vi "LinVer Protokoll_Daten.vi"(9 "Lin-Polynom":T4={"Messgerät"="", "Kalibrator (Gasteiler)"="", "Bearbeiter/in"="", "Komponente"="", "Zeitstempel"=timestamp(0 s since 1904-01-01), "F_max gefordert (%)"=0.0, "F_max in %"=0.0, "F_max in ppm"=0.0, "Vorschlag Ordnung"=0, "Polynom OK"=FALSE, "Polynomkoeff."=[], "Prüfgas Konzentration"=0.0, "Pfad EPA"="", "Pfad_LIN"="", "Gasnummer:"=0, "Komponentenauswahl"=[], "Verdünnungsgas"=0, "Zeitdauer Stufe"=0.0, "Anzahl Stufen"=0.0, "F_max in % EPA"=0.0, "F_max in ppm EPA"=0.0, "F_max in % LIN"=0.0, "F_max in ppm LIN"=0.0, "Punkte umkehren"=FALSE, "EPA Optionsfeld"=enum."Rohwert", "Autolin Hovacal"=enum."Optionsauswahl 2", "Spanfactors"=[], "Kalibrierauswahl"=0, "Conditions:"=0, "Gasflaschen Nr.:"="", "Bottle Accuracy"=0.0, "Konfig Gasflasche"=FALSE, "Gasflasche"=0, "HovaCAL Flow AutoLin"={"HovaCAL Flow Input Cluster"=0.0}, "MFC Output"={"Run"=FALSE}, "Gas Ablaufdatum"=timestamp(0 s since 1904-01-01), "Lin Modus"=0, "zusätzliche Zeitdauer Erster Punkt"=0.0, "Offsets"=[]} {"zusätzliche Zeitdauer Erster Punkt" format="%#_5g"; "Lin Modus" items=["Cal Gas to PNS", "Cal Gas to Samplepoint", "Measure"]; "Gas Ablaufdatum" format="%<%d.%m.%Y>T"; "HovaCAL Flow AutoLin"."HovaCAL Flow Input Cluster" format="%.2f"; "Gasflasche" items=["----"=10000, "IAG MG"=0, "IAG NH3 3000"=1, "IAG NH3 2000"=2, "IAG NH3 200"=3]; "Conditions:" items=["field", "laboratory"]; "Kalibrierauswahl" items=["Inaktiv", "Aktiv"]; "Anzahl Stufen" format="%#_5g"; "Zeitdauer Stufe" format="%#_5g"; "Verdünnungsgas" items=["N2", "O2"]; "Komponentenauswahl"."Konzentration" format="%#.6f"; "Gasnummer:" min=1 max=5; "Prüfgas Konzentration" format="%#.6f"; "Polynomkoeff." format="%#_18f"}, 10 "Aktiv":T1, 11 "Eingabetabelle":T3) -> (0 "EPA Auswertung":cluster{sgl[], sgl[], bool[]}, 1 "Ausgangs-Cluster":T4={"Messgerät"="", "Kalibrator (Gasteiler)"="", "Bearbeiter/in"="", "Komponente"="", "Zeitstempel"=timestamp(0 s since 1904-01-01), "F_max gefordert (%)"=0.0, "F_max in %"=0.0, "F_max in ppm"=0.0, "Vorschlag Ordnung"=0, "Polynom OK"=FALSE, "Polynomkoeff."=[], "Prüfgas Konzentration"=0.0, "Pfad EPA"="", "Pfad_LIN"="", "Gasnummer:"=0, "Komponentenauswahl"=[], "Verdünnungsgas"=0, "Zeitdauer Stufe"=0.0, "Anzahl Stufen"=0.0, "F_max in % EPA"=0.0, "F_max in ppm EPA"=0.0, "F_max in % LIN"=0.0, "F_max in ppm LIN"=0.0, "Punkte umkehren"=FALSE, "EPA Optionsfeld"=enum."Rohwert", "Autolin Hovacal"=enum."Optionsauswahl 2", "Spanfactors"=[], "Kalibrierauswahl"=0, "Conditions:"=0, "Gasflaschen Nr.:"="", "Bottle Accuracy"=0.0, "Konfig Gasflasche"=FALSE, "Gasflasche"=0, "HovaCAL Flow AutoLin"={"HovaCAL Flow Input Cluster"=0.0}, "MFC Output"={"Run"=FALSE}, "Gas Ablaufdatum"=timestamp(0 s since 1904-01-01), "Lin Modus"=0, "zusätzliche Zeitdauer Erster Punkt"=0.0, "Offsets"=[]} {"zusätzliche Zeitdauer Erster Punkt" format="%#_5g"; "Lin Modus" items=["Cal Gas to PNS", "Cal Gas to Samplepoint", "Measure"]; "Gas Ablaufdatum" format="%<%d.%m.%Y>T"; "HovaCAL Flow AutoLin"."HovaCAL Flow Input Cluster" format="%.2f"; "Gasflasche" items=["----"=10000, "IAG MG"=0, "IAG NH3 3000"=1, "IAG NH3 2000"=2, "IAG NH3 200"=3]; "Conditions:" items=["field", "laboratory"]; "Kalibrierauswahl" items=["Inaktiv", "Aktiv"]; "Anzahl Stufen" format="%#_5g"; "Zeitdauer Stufe" format="%#_5g"; "Verdünnungsgas" items=["N2", "O2"]; "Komponentenauswahl"."Konzentration" format="%#.6f"; "Gasnummer:" min=1 max=5; "Prüfgas Konzentration" format="%#.6f"; "Polynomkoeff." format="%#_18f"}, 2 "Auswertung Daten":string[](array[string]), 3 "Tabelle":T3)   [LabVIEW 2020, in "Linearisierung v2.lvlib" / "Linearity verification 1065-307.lvlib"]
uses:
  Linearity verification 1065-307.lvlib
  Lin-Polynom Daten.ctl
  KomponentenArray.ctl
  Visualisierungs Elemente/Auswahlfeld.ctl
  Visualisierungs Elemente/Zahlen-Eingabefeld.ctl
  EPA Optionsfeld.ctl
  Gasteiler/HovaCal/AutoLin Hovacal.ctl
  Kalibrieroption.ctl
  Condition.ctl
  Seiten/System Einstellungen V2/Konfig Gasflasche.ctl
  Seiten/System Einstellungen V2/Gasflasche Auswahl.ctl
  Gasteiler/HovaCAL_Interface/Controls/Flow Einstellung.ctl
  Gasteiler/HovaCAL_Interface/Controls/Pump state.ctl
  Seiten/CalGas Aufschaltung/Lin Modus.ctl
  Eingabetabelle.ctl
  AktivArray.ctl
  AktivButton.ctl
  Sprachverwaltung/FGV Aktion Tabelle zerlegen.ctl
  Sprachverwaltung/Sprachverwaltung.lvlib
  AutoLin Protokoll/AutoLin Protokoll.lvlib
  Linearisierung v2.lvlib
  Allgemein/allgemeine Sub-VIs.lvlib
  Gasteiler/Gasteiler.lvlib
  Gasteiler/HovaCal/HovaCal.lvlib
  Seiten/System Einstellungen V2/System Einstellungen V2.lvlib
  Gasteiler/HovaCAL_Interface/Controls/Controls.lvlib
  Seiten/CalGas Aufschaltung/CalGas Aufschaltung.lvlib
panel:
  # "Tabelle:\n0.....Sollwert\n1.....Istwert\n2.....Rohwert\n3.....linearisiert\n4.....abs.Fehler ppm\n5.....Fehler in %\n6.....Deviation\n7.....Temp.Messzelle\n8.....Druck Messzelle\n9.....abs.Fehler ppm linearisiert\n10....Fehler in % linearisiert\n11....abs.Fehler ppm EPA\n12....Fehler in % EPA\n13....abs.Fehler ppm Rohwert\n14....Fehler in % Rohwert"
  # "%"
  # "%"
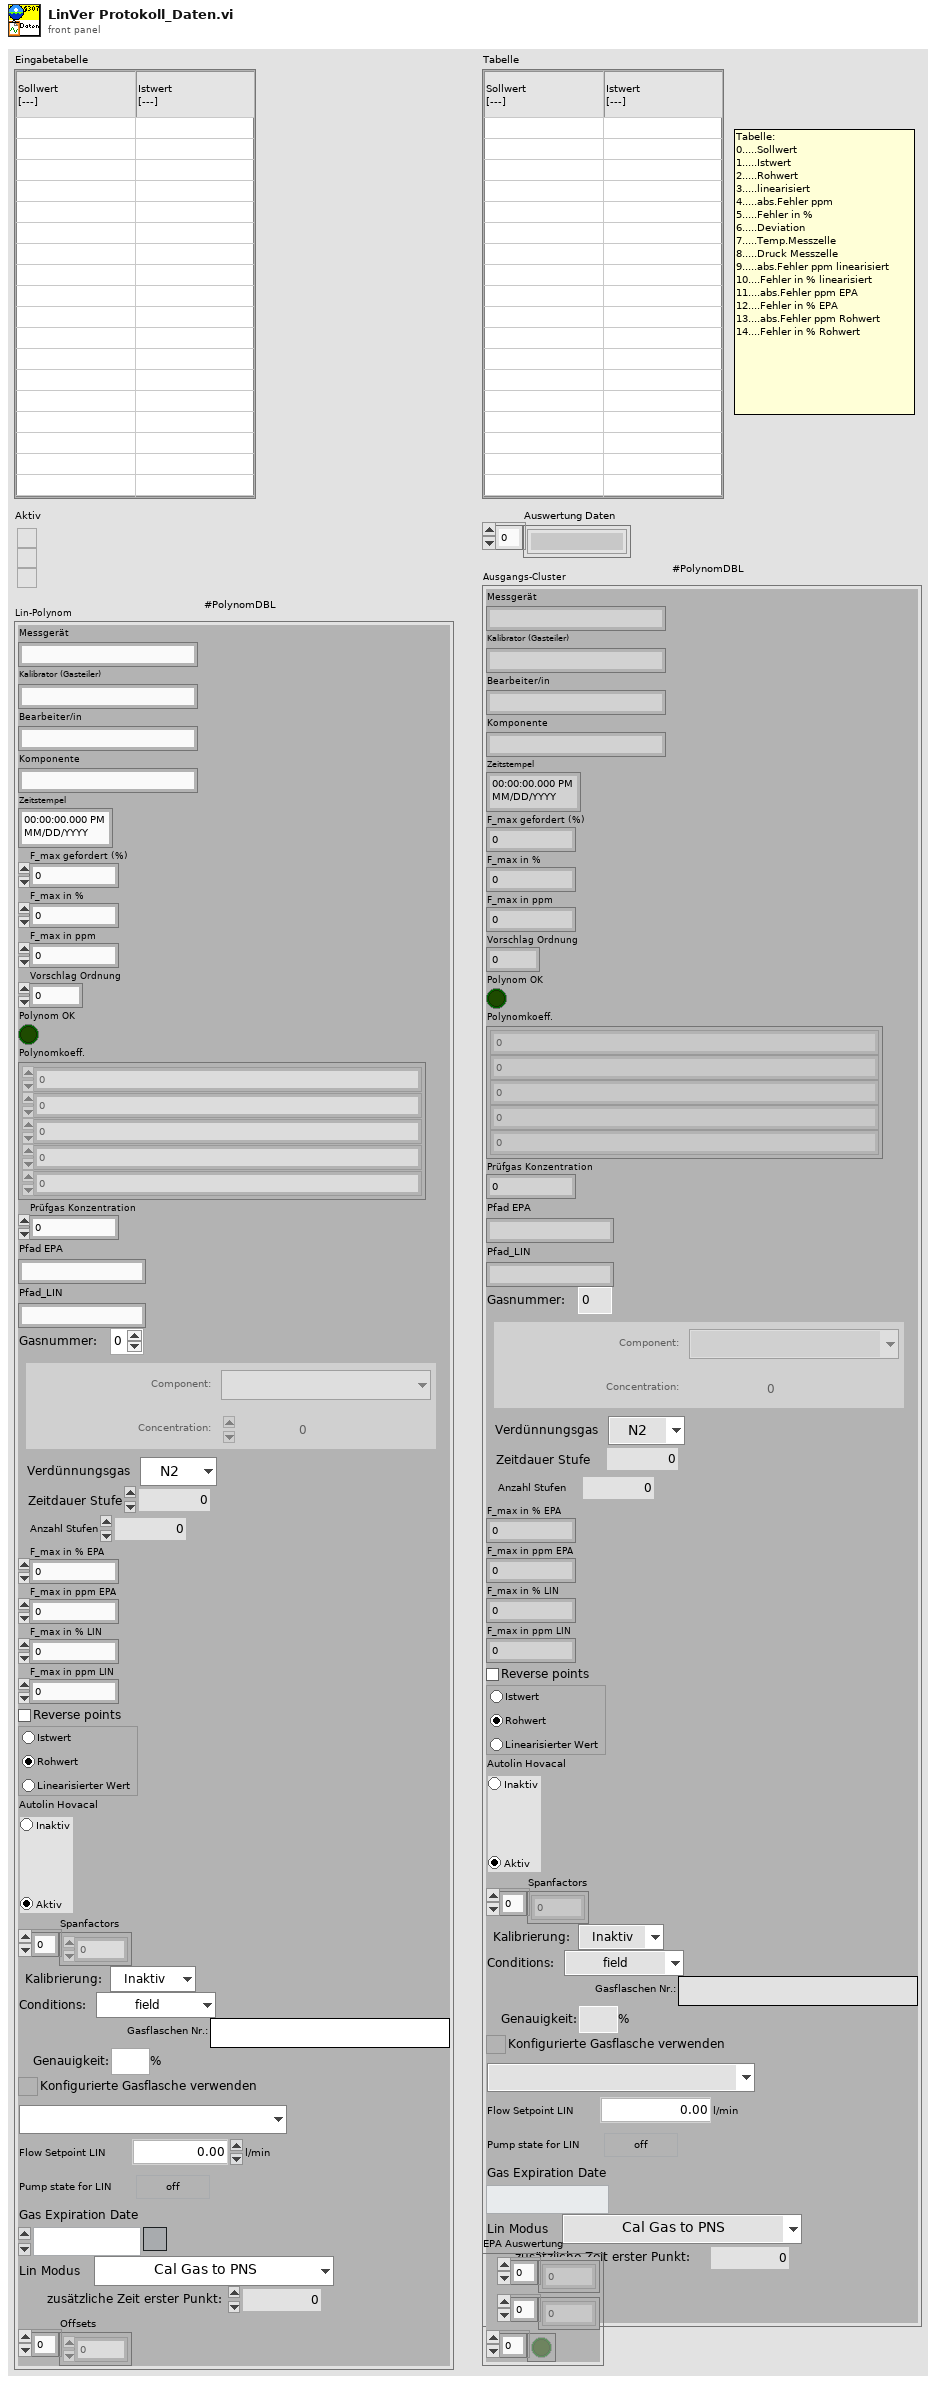
[diagram p1: front panel]
types:
  T1 = typedef "Linearisierung v2.lvlib/AktivArray.ctl" = T2[]
  T2 = typedef "Linearisierung v2.lvlib/AktivButton.ctl" = bool
  T3 = typedef "Linearisierung v2.lvlib/Eingabetabelle.ctl" = string[][]
  T4 = typedef "Linearisierung v2.lvlib/Lin-Polynom Daten.ctl" = cluster{"Messgerät":string, "Kalibrator (Gasteiler)":string, "Bearbeiter/in":string, "Komponente":string, "Zeitstempel":timestamp, "F_max gefordert (%)":sgl, "F_max in %":sgl, "F_max in ppm":sgl, "Vorschlag Ordnung":i32, "Polynom OK":bool, "Polynomkoeff.":dbl[], "Prüfgas Konzentration":dbl, "Pfad EPA":string, "Pfad_LIN":string, "Gasnummer:":u8, "Komponentenauswahl":T5, "Verdünnungsgas":T7, "Zeitdauer Stufe":T8, "Anzahl Stufen":T8, "F_max in % EPA":sgl, "F_max in ppm EPA":sgl, "F_max in % LIN":sgl, "F_max in ppm LIN":sgl, "Punkte umkehren":bool, "EPA Optionsfeld":T9, "Autolin Hovacal":T10, "Spanfactors":sgl[], "Kalibrierauswahl":T11, "Conditions:":T12, "Gasflaschen Nr.:":string, "Bottle Accuracy":dbl, "Konfig Gasflasche":T13, "Gasflasche":T14, "HovaCAL Flow AutoLin":T15, "MFC Output":T16, "Gas Ablaufdatum":timestamp, "Lin Modus":T17, "zusätzliche Zeitdauer Erster Punkt":sgl, "Offsets":sgl[]}
  T5 = typedef "Linearisierung v2.lvlib/KomponentenArray.ctl" = cluster{"Komponente:":T6, "Konzentration":dbl}[]
  T6 = typedef "Auswahlfeld.ctl" = u16
  T7 = typedef "Linearisierung v2.lvlib/Gasteiler.lvlib/Prüfgas in.ctl" = u16
  T8 = typedef "Zahlen-Eingabefeld.ctl" = sgl
  T9 = typedef "Linearisierung v2.lvlib/EPA Optionsfeld.ctl" = enum32{"Istwert", "Rohwert", "Linearisierter Wert"}
  T10 = typedef "Linearisierung v2.lvlib/Gasteiler.lvlib/HovaCal.lvlib/AutoLin Hovacal.ctl" = enum32{"Keine Auswahl", "Optionsauswahl 1", "Optionsauswahl 2"}
  T11 = typedef "Linearisierung v2.lvlib/Kalibrieroption.ctl" = u16
  T12 = typedef "Linearisierung v2.lvlib/Linearity verification 1065-307.lvlib/Condition.ctl" = u16
  T13 = typedef "System Einstellungen V2.lvlib/Konfig Gasflasche.ctl" = bool
  T14 = typedef "System Einstellungen V2.lvlib/Gasflasche Auswahl.ctl" = u16
  T15 = typedef "Linearisierung v2.lvlib/Gasteiler.lvlib/HovaCAL_Interface.lvlib/Controls.lvlib/Flow Einstellung.ctl" = cluster{"HovaCAL Flow Input Cluster":dbl}
  T16 = typedef "Linearisierung v2.lvlib/Gasteiler.lvlib/HovaCAL_Interface.lvlib/Controls.lvlib/Pump state.ctl" = cluster{"Run":bool}
  T17 = typedef "CalGas Aufschaltung.lvlib/Lin Modus.ctl" = u16
  T18 = typedef "Sprachverwaltung.lvlib/FGV Aktion Tabelle zerlegen.ctl" = enum16{"laden", "vereinzeln", "speichern"}
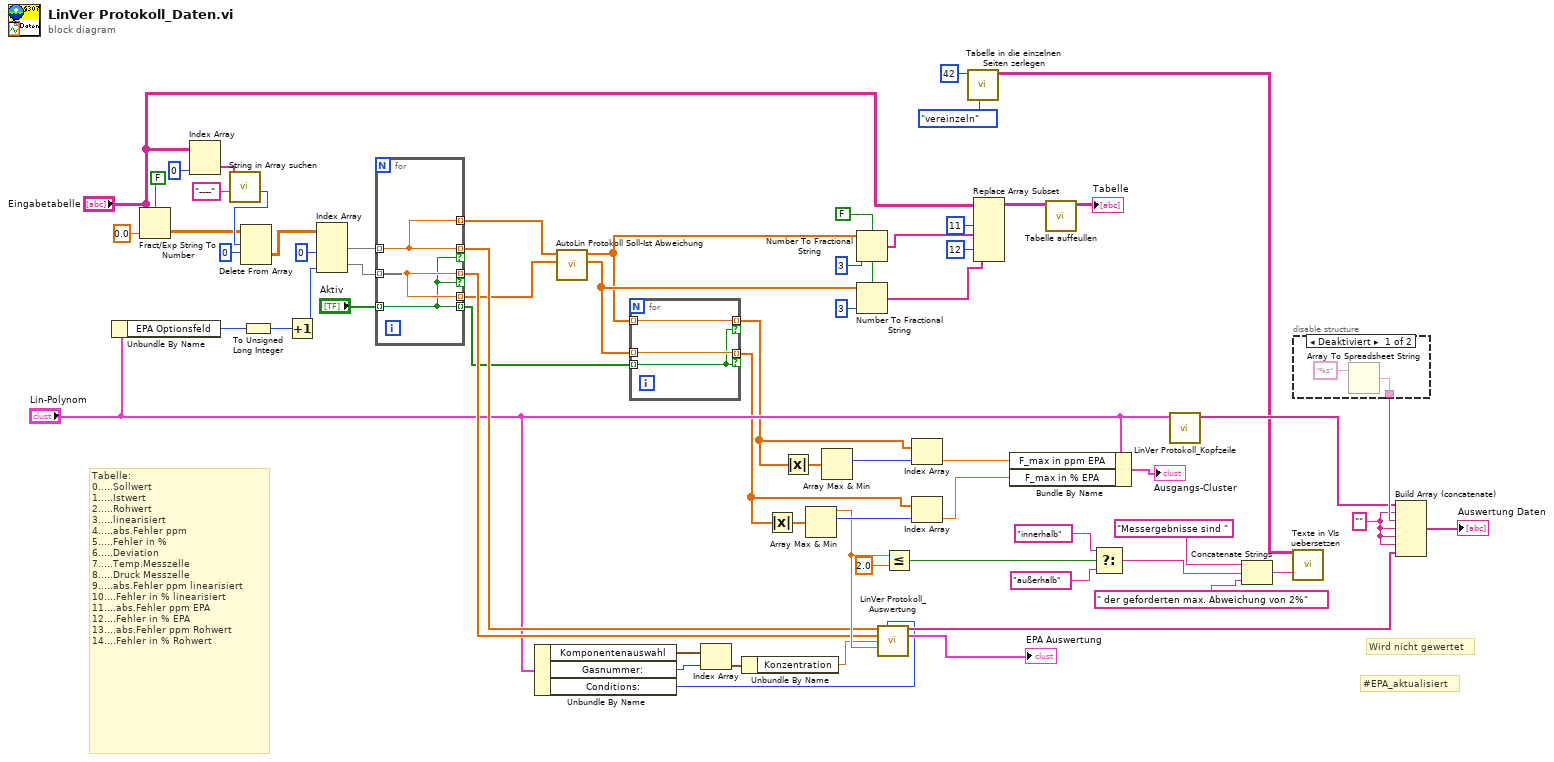
[diagram p0: block diagram]
diagram:
  w3 = FALSE ("Systemdezimalzeichen verwenden (T)")
  w44 = ""
  # "Tabelle:\n0.....Sollwert\n1.....Istwert\n2.....Rohwert\n3.....linearisiert\n4.....abs.Fehler ppm\n5.....Fehler in %\n6.....Deviation\n7.....Temp.Messzelle\n8.....Druck Messzelle\n9.....abs.Fehler ppm linearisiert\n10....Fehler in % linearisiert\n11....abs.Fehler ppm EPA\n12....Fehler in % EPA\n13....abs.Fehler ppm Rohwert\n14....Fehler in % Rohwert"
  # "#EPA_aktualisiert"
  # "Wird nicht gewertet"
  n1 = Unbundle By Name("Lin-Polynom") -> ("EPA Optionsfeld"=w13:T9)
  n2 = Fract/Exp String To Number(use system decimal point (T)=FALSE ("Systemdezimalzeichen verwenden (T)"), string="Eingabetabelle", default (0 dbl)=0.0) -> (number=w17:dbl[][])  [unwired: 1 in, 1 out]
  n3 = Index Array(array="Eingabetabelle", index (col)=0 ("Deaktivierter Index (Spalte)")) -> (element=w20:string[])  [unwired: 1 in]
  n4 = call "String in Array suchen.vi"("Nach String/Zeichen suchen (-)"="----", "String-Array"=w20) -> ("Index"=w21:i32)  [unwired: 7 in, 2 out]
  n5 = Delete From Array(array=w17, length=w21, index (row)=0 ("Index (Zeile)")) -> (deleted portion=w16:dbl[][])  [unwired: 1 in, 1 out]
  n6 = To Unsigned Long Integer(number=w13) -> (unsigned 32bit integer=w12:u32)
  n7 = Increment(x=w12) -> (x+1=w11:u32)
  n8 = Index Array(array=w16, index (col) #1=0 ("Deaktivierter Index (Spalte)"), index (col) #2=w11) -> (element #1=w30:dbl[], element #2=w29:dbl[])  [unwired: 2 in]
  n9 = for {
    tunnel: w30 -> [w69] mode=indexing
    tunnel: w29 -> [w68] mode=indexing
    tunnel: [w69] -> w27 mode=indexing if=w67
    tunnel: [w68] -> w26 mode=indexing if=w67
    tunnel: "Aktiv" -> [w67] mode=indexing
    tunnel: [w69] -> w10 mode=indexing
    tunnel: [w68] -> w9 mode=indexing
    tunnel: [w67] -> w7 mode=indexing
  }
  n10 = Unbundle By Name("Lin-Polynom") -> ("Komponentenauswahl"=w35:T5, "Gasnummer:"=w32:u8, "Conditions:"=w1:T12)
  n11 = call "AutoLin Protokoll Soll-Ist Abweichung.vi"("Istwerte (ppm)"=w9, "Sollwerte (ppm)"=w10) -> ("% vom Sollwert"=w8:sgl[], "abs. Fehler (ppm)"=w5:sgl[])  [unwired: 7 in, 1 out]
  n12 = for {
    tunnel: w8 -> [w72] mode=indexing
    tunnel: w7 -> [w70] mode=indexing
    tunnel: [w72] -> w6 mode=indexing if=w70
    tunnel: w5 -> [w71] mode=indexing
    tunnel: [w71] -> w4 mode=indexing if=w70
  }
  n13 = Index Array(array=w35, index=w32) -> (element=w34:cluster{"Komponente:":T6, "Konzentration":dbl})
  n14 = Unbundle By Name(w34) -> ("Konzentration"=w33:dbl)
  n15 = Absolute Value(x=w6) -> (abs(x)=w63:sgl[])
  n16 = Absolute Value(x=w4) -> (abs(x)=w62:sgl[])
  n17 = Array Max & Min(array=w63) -> (max value=w48:sgl, max index (indices)=w66:i32)  [unwired: 2 out]
  n18 = Array Max & Min(array=w62) -> (max index (indices)=w65:i32)  [unwired: 3 out]
  n19 = Number To Fractional String(use system decimal point (T)=w3, number=w5, precision (6)=i16 3 ("Genauigkeit (6)")) -> (F-format string=w39:string[])  [unwired: 1 in]
  n20 = Number To Fractional String(use system decimal point (T)=w3, number=w8, precision (6)=i16 3 ("Genauigkeit (6)")) -> (F-format string=w38:string[])  [unwired: 1 in]
  n21 = call "LinVer Protokoll_Auswertung.vi"("Sollwerte"=w27, "Bedingung:"=w1, "Istwerte"=w26, "Konzentration"=w33, "Maximale Abweichung"=w48) -> (4:"Auswertung"=w53:string[], 6:"Auswertung"=→"EPA Auswertung":cluster{sgl[], sgl[], bool[]})  [unwired: 8 in, 1 out]
  n22 = Less Or Equal?(x=w48, y=sgl 2.0) -> (x <= y?=w50:bool)
  n23 = Index Array(array=w4, index=w65) -> (element=w64:sgl)
  n24 = Index Array(array=w6, index=w66) -> (element=w51:sgl)
  n25 = call "Tabelle in die einzelnen Seiten zerlegen.vi"("Aktion"=FGV_Aktion_Tabelle_zerlegen."vereinzeln", "Index (Seite)"=42) -> ("Sprachliste"=w45:string[][])  [unwired: 7 in, 2 out]
  n26 = Replace Array Subset(array="Eingabetabelle", new element #1=w39, index (col) #1=11 ("Deaktivierter Index (Spalte)"), new element #2=w38, index (col) #2=12 ("Index (Spalte)")) -> (w25:T3)  [unwired: 2 in]
  n27 = Bundle By Name(cluster="Lin-Polynom", "F_max in ppm EPA"=w64, "F_max in % EPA"=w51) -> (→"Ausgangs-Cluster":T4)
  n28 = call "Tabelle auffeullen.vi"("Neue Tabelle"=w25) -> ("Tabelle"=→"Tabelle":string[][])  [unwired: 10 in]
  n29 = Select(t="innerhalb", s=w50, f="außerhalb") -> (s? t:f=w55:string)
  n30 = call "LinVer Protokoll_Kopfzeile.vi"("Protokolldaten"="Lin-Polynom") -> ("Protokollkopf"=w52:string[])  [unwired: 9 in, 1 out]
  n31 = Concatenate Strings("Messergebnisse sind ", w55, " der geforderten max. Abweichung von 2%") -> (w46:string)
  n32 = call "Texte in VIs uebersetzen.vi"("Sprachliste"=w45, "String zum Übersetzen"=w46) -> ()  [unwired: 9 in, 5 out]
  n33 = disable-structure shown="Deaktiviert" {
    disable-tunnel: [w73 _] -> w61
    frame Disabled {
      n34 = Array To Spreadsheet String(3:"%s" ("Format-String")) -> (spreadsheet string=w73:string)  [unwired: 2 in]
    }
    frame Enabled {
    }
  }
  n35 = Build Array (concatenate)(w52, w44, w61, w44, w44, w44, w53) -> (→"Auswertung Daten":string[])
